vi "Set or Get ActiveCell Justify.vi"(8 "error in (no error)":errorcluster caption="错误输入（无错误）", 9 "Mode":T1, 10 "Justify In":enum16{"Left", "Center", "Right"}(ring), 11 "Table Ref In":refnum<vi>) -> (0 "error out":errorcluster caption="错误输出", 2 "Justify Out":enum16{"Left", "Center", "Right"}(ring), 3 "Table Ref Out":refnum<vi>)   [LabVIEW 2012, in "Table Tool.lvlib"]
uses:
  GetOrSet.ctl
  Table Tool.lvlib
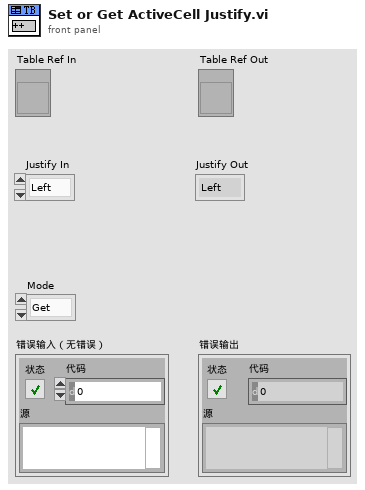
[diagram p1: front panel]
types:
  T1 = typedef "Table Tool.lvlib/GetOrSet.ctl" = enum16{"Get", "Set"}
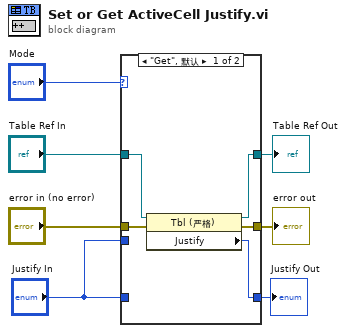
[diagram p0: block diagram]
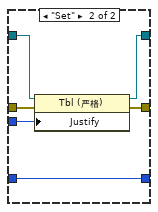
[diagram p2: hidden frame]
diagram:
  n1 = case shown="\"Get\", 默认" "Mode" {
    tunnel: "Table Ref In" -> [w12 w17]
    tunnel: "error in (no error)" -> [w11 w18]
    tunnel: [w10 w15] -> w4
    tunnel: [w9 w16] -> w3
    tunnel: "Justify In" -> [_ w14]
    tunnel: "Justify In" -> [_ w13]
    tunnel: [w8 w13] -> w1
    frame "Get", Default {
      n2 = property class="Tbl (严格)"(reference=w12, error in=w11) -> (reference out=w9:refnum<vi>, error out=w10:errorcluster, "Justify"=w8:enum16{"Left", "Center", "Right"})
    }
    frame "Set" {
      n3 = property class="Tbl (严格)"(reference=w17, error in=w18, "Justify"=w14) -> (reference out=w16:refnum<vi>, error out=w15:errorcluster)
    }
  }
  "Table Ref Out" <- w3
  "error out" <- w4
  "Justify Out" <- w1
